vi "FindStartEndPointsRRTImproved.vi"(4 "ignoreBall?":bool, 5 "Robot in":T1={"id"=0, "function"=enum."Attacker", "x"=0.0, "y"=0.0, "orientation"=0.0, "v_tangent"=0.0, "v_normal"=0.0, "v_ang"=0.0, "kick_x"=0.0, "kick_z"=0.0, "dribble"=FALSE, "Timestamp"=timestamp(0 s since 1904-01-01), "estimatives"={"est_v_tangent"=0.0, "est_v_normal"=0.0, "est_vx"=0.0, "est_vy"=0.0, "Pos Robot Est"=[]}, "dest_x_kick"=0.0, "dest_y_kick"=0.0, "Gap Coord"=[], "States"=enum."Pass", "Path "=[], "Path  Smooth"=[], "Dest"=[], "vx_desired"=0.0, "vy_desired"=0.0, "slowBehavior"=FALSE, "VSSStates"=enum."Pass"}, 6 "enemy_robots":T1[](array[typedef]), 7 "ball":dbl[](array[numeric]), 8 "our_robots":T1[](array[typedef]), 9 "Goal":dbl[](array[numeric]), 10 "Initial State":dbl[](array[numeric]), 11 "Collision Points":dbl[][](array[numeric])) -> (2 "Start End Points RRT":dbl[][](array[numeric]))   [LabVIEW 2020]
uses:
  Vision_class/Old vision/Controls/AI Robot.ctl
  Vision_class/Old vision/Controls/Functions Enum.ctl
  Vision_class/Old vision/Controls/AttackerStates.ctl
  Vision_class/Old vision/Controls/PathDests.ctl
  Vision_class/Old vision/Controls/PathDest.ctl
  Navigation/VSSNavigation/VSSAttackerStates.ctl
  <vilib>/Analysis/_algsub.llb/Real Vector Norm.vi
  <vilib>/Analysis/NI_AALPro.lvlib
panel:
  in  "tamanho minimo":dbl=300.0 format="%#_13g"
  in  "threshold":dbl=100.0 format="%#_13g"
  out "Collision Points \nordenado":dbl[][](array[numeric])
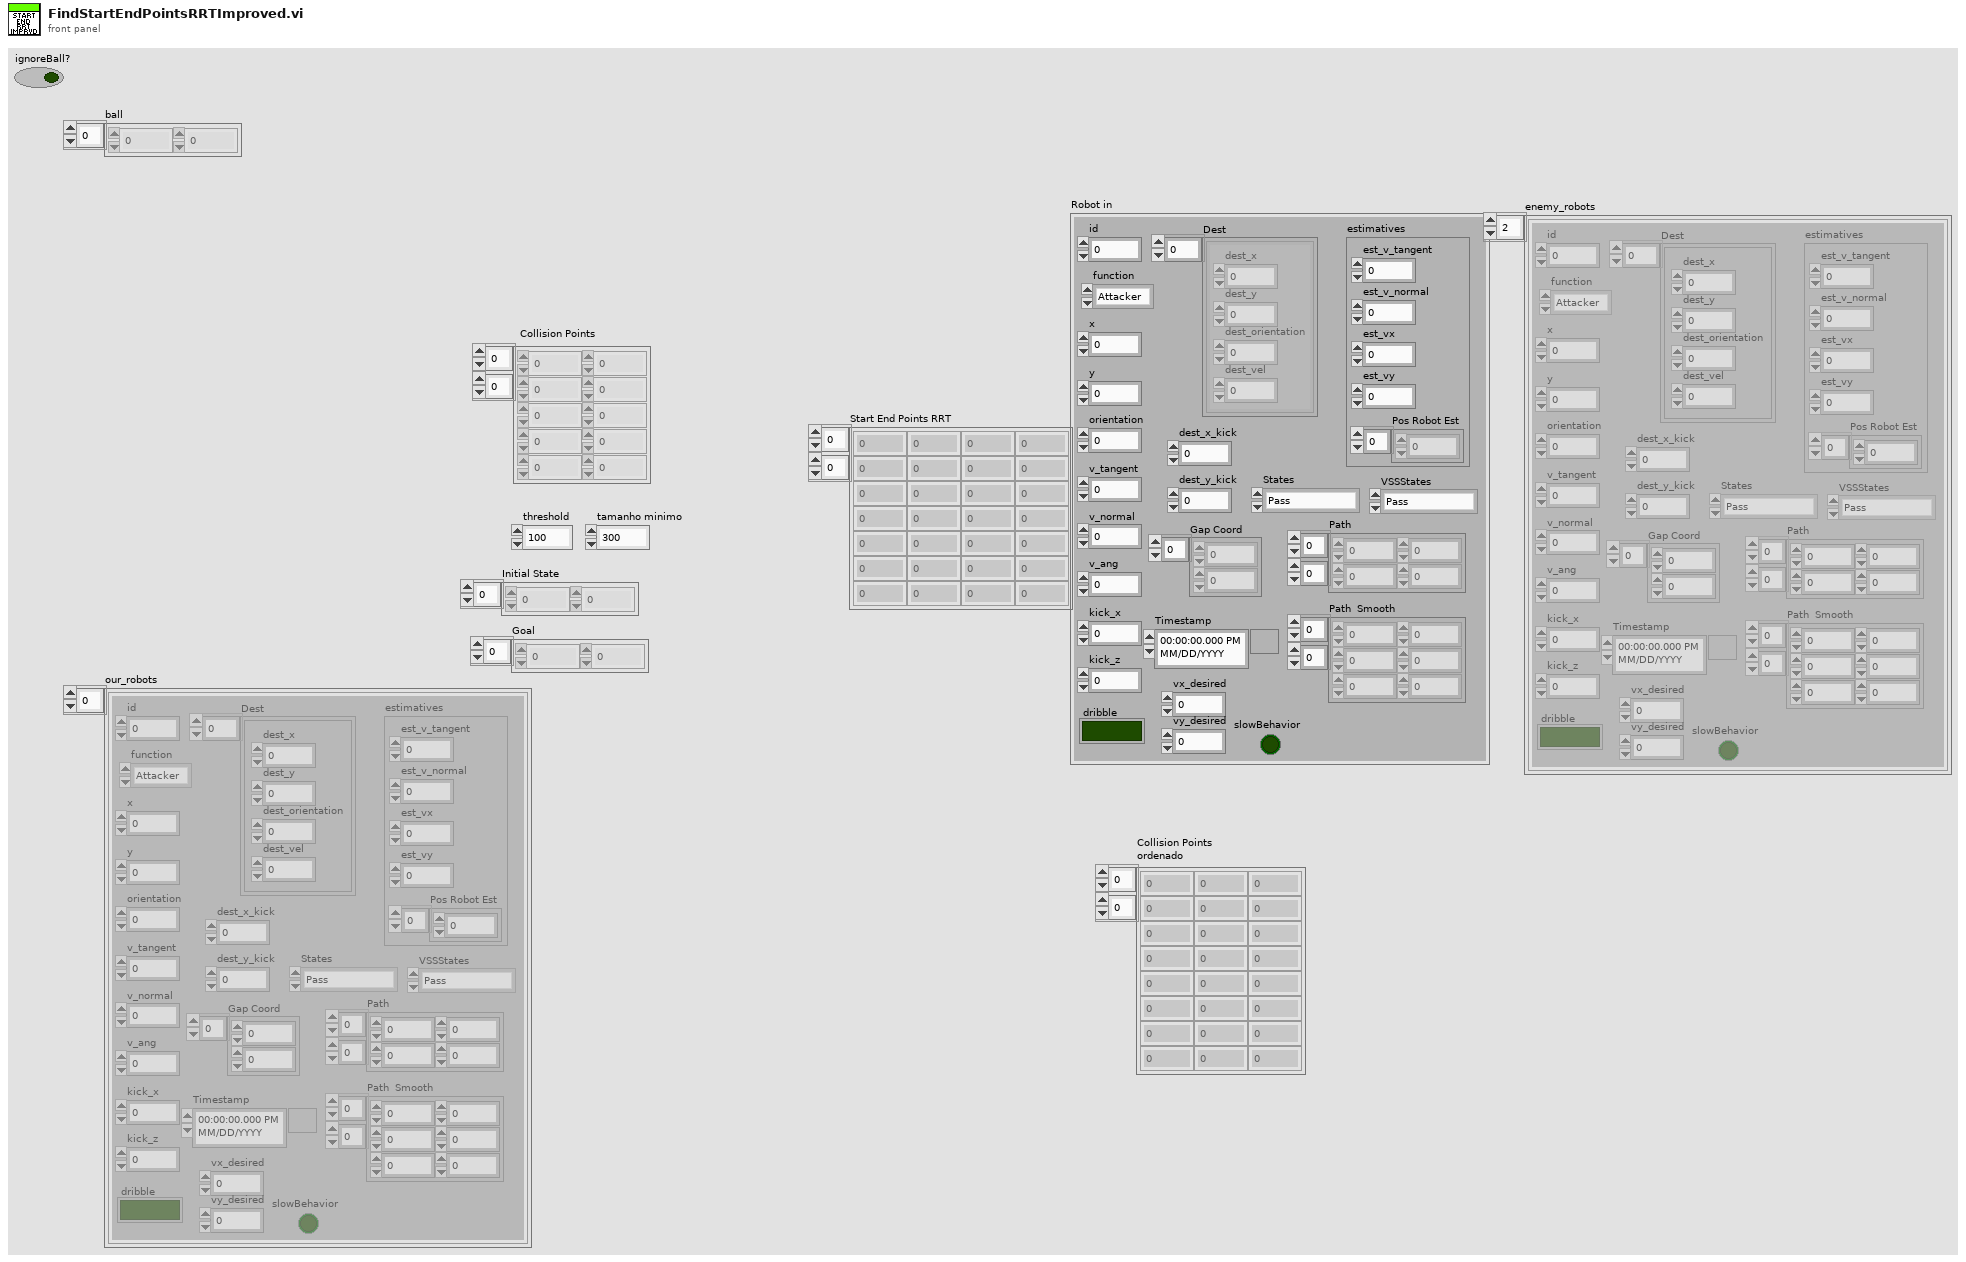
[diagram p1: front panel]
types:
  T1 = typedef "AI Robot.ctl" = cluster{"id":u32, "function":T2, "x":dbl, "y":dbl, "orientation":dbl, "v_tangent":dbl, "v_normal":dbl, "v_ang":dbl, "kick_x":dbl, "kick_z":dbl, "dribble":bool, "Timestamp":timestamp, "estimatives":cluster{"est_v_tangent":dbl, "est_v_normal":dbl, "est_vx":dbl, "est_vy":dbl, "Pos Robot Est":dbl[]}, "dest_x_kick":dbl, "dest_y_kick":dbl, "Gap Coord":dbl[], "States":T3, "Path ":dbl[][], "Path  Smooth":dbl[][], "Dest":T4, "vx_desired":dbl, "vy_desired":dbl, "slowBehavior":bool, "VSSStates":T6}
  T2 = typedef "Functions Enum.ctl" = enum16{"2nd Striker", "Attacker", "Goalie", "Defender", "Striker", "Goto 0", "Dummy", "Kicker", "ZigZag 0", "ZigZag 1", "ZigZag 2", "ZigZag 3", "ZigZag 4", "ZigZag 5", "ZigZag 6", "ZigZag 7", "ZigZag 8", ""}
  T3 = typedef "AttackerStates.ctl" = enum16{"Pass", "GoToTangent", "BallGetting", "GoToKick", ""}
  T4 = typedef "PathDests.ctl" = T5[]
  T5 = typedef "PathDest.ctl" = cluster{"dest_x":dbl, "dest_y":dbl, "dest_orientation":dbl, "dest_vel":dbl}
  T6 = typedef "VSSAttackerStates.ctl" = enum16{"Pass", "GoToTangent", "BallGetting", "GoToKick", "Rotate anti-clockwise", "Rotate Clockwise", ""}
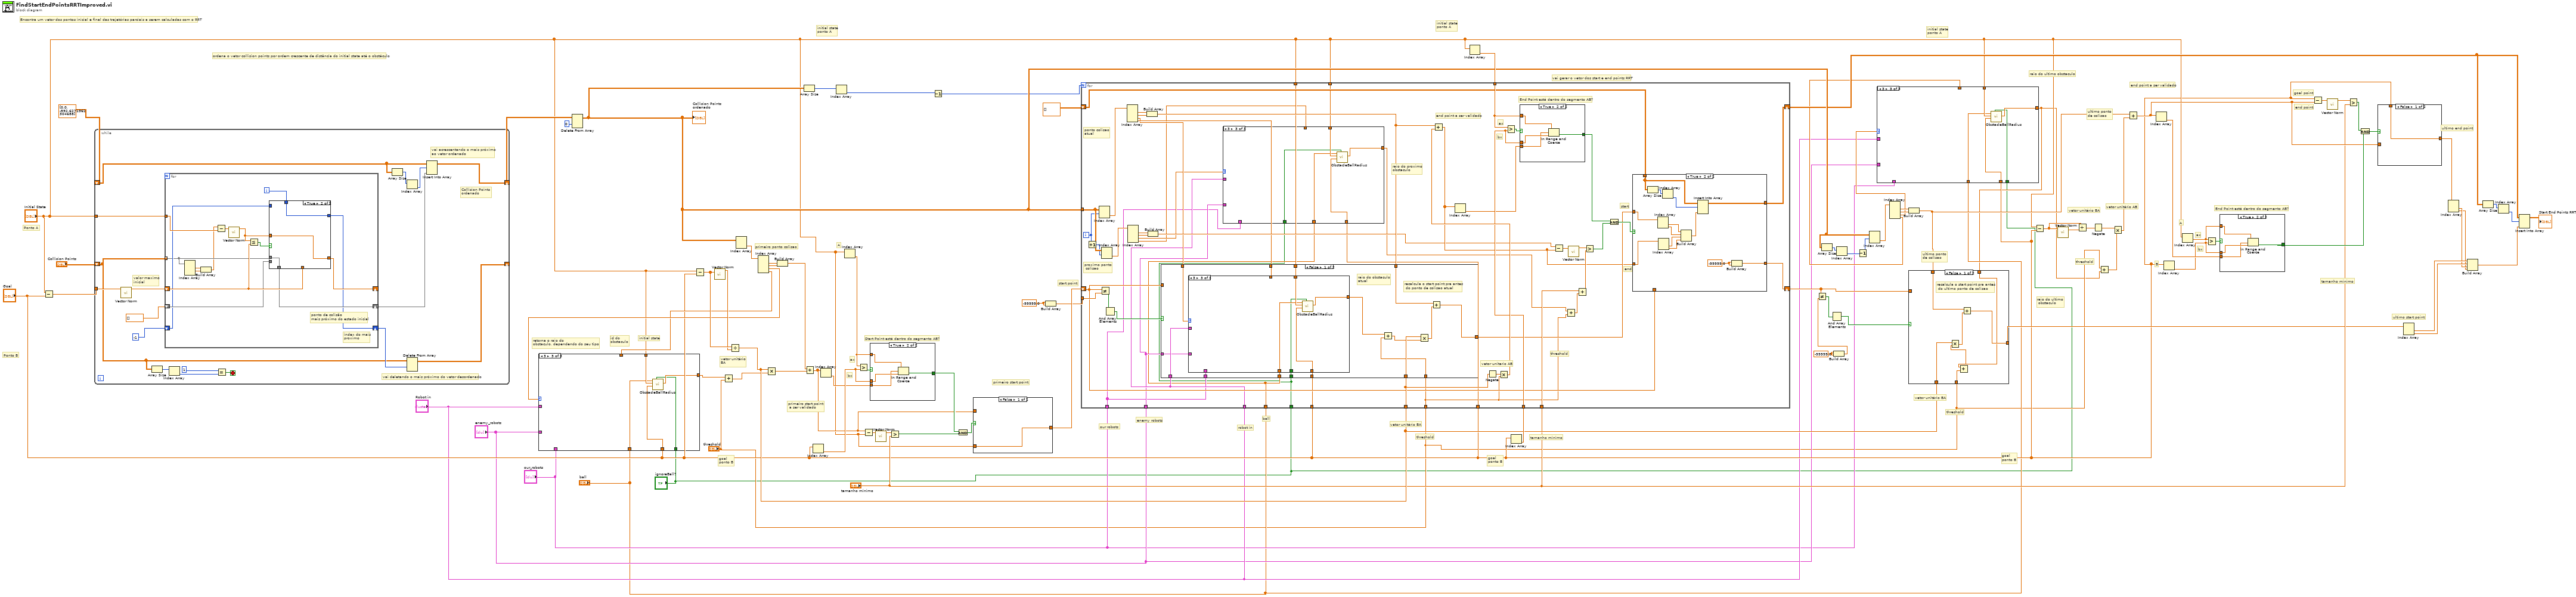
[diagram p0: block diagram]
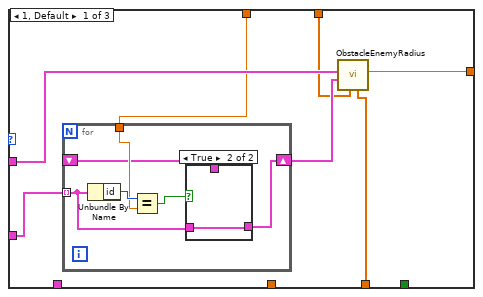
[diagram p2: hidden frame]
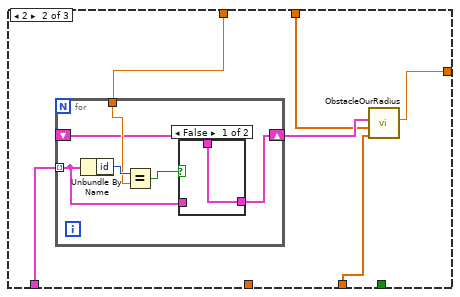
[diagram p4: hidden frame]
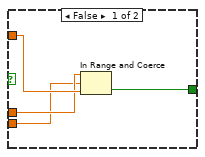
[diagram p6: hidden frame]
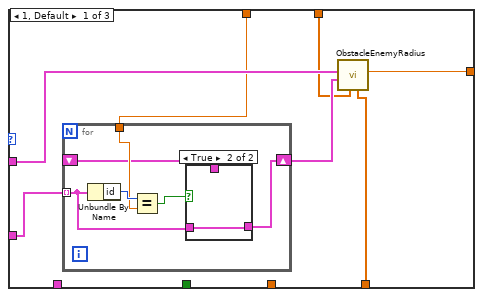
[diagram p9: hidden frame]
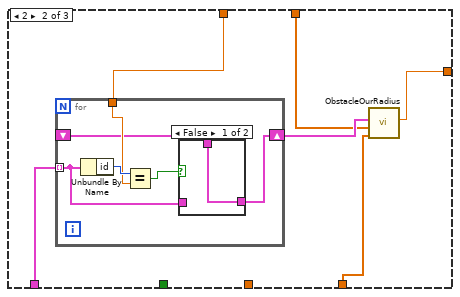
[diagram p11: hidden frame]
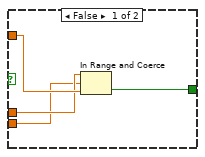
[diagram p14: hidden frame]
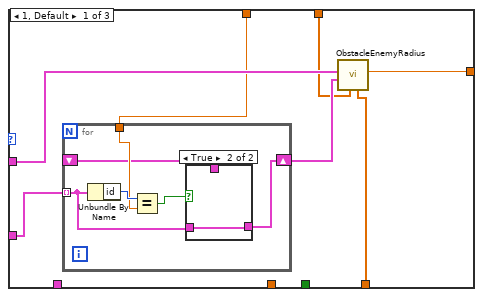
[diagram p15: hidden frame]
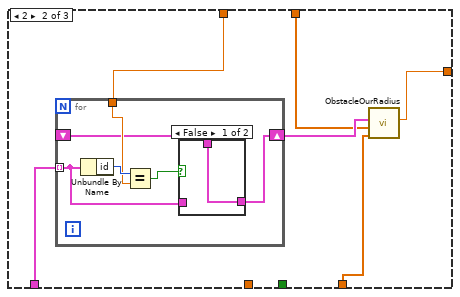
[diagram p17: hidden frame]
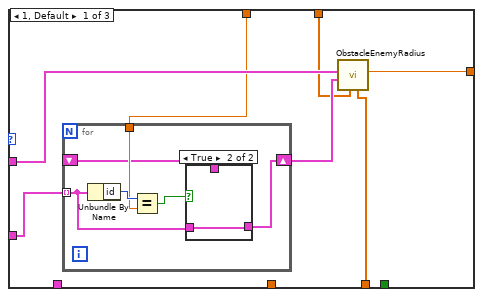
[diagram p20: hidden frame]
diagram:
  w47 = -99999.0 ("element")
  w52 = -99999.0 ("element")
  # "raio do ultimo\n obstaculo"
  # "raio do ultimo obstaculo"
  # "ball"
  # "robot in"
  # "enemy robots"
  # "our robots"
  # "initial state"
  # "id do\nobstaculo"
  # "retorna o raio do \nobstaculo, dependendo do seu tipo"
  # "vai gerar o vetor dos start e end points RRT"
  # "ultimo start point"
  # "ultimo end point"
  # "tamanho minimo"
  # "end point a ser validado"
  # "ultimo ponto\nde colisao"
  # "threshold"
  # "goal\nponto B"
  # "initial state\nponto A"
  # "ultimo ponto\nde colisao"
  # "threshold"
  # "vetor unitário BA"
  # "tamanho minimo"
  # "initial state\nponto A"
  # "goal\nponto B"
  # "threshold"
  # "vetor unitário BA"
  # "start point"
  # "primeiro start point"
  # "A"
  # "Start Point está dentro do segmento AB?"
  # "bx"
  # "ax"
  # "primeiro start point\n a ser validado"
  # "primeiro ponto colisao"
  # "vetor unitário\nBA"
  # "initial state\nponto A"
  # "goal\nponto B"
  # "ordena o vetor collision points por ordem crescente de distância do initial state até o obstáculo"
  # "Encontra um vetor dos pontos inicial e final das trajetórias parciais a serem calculadas com o RRT"
  # "end point"
  # "goal point"
  # "End Point está dentro do segmento AB?"
  # "bx"
  # "ax"
  # "B"
  # "A"
  # "vetor unitário AB"
  # "vetor unitário BA"
  # "Ponto B"
  # "Ponto A"
  n1 = Subtract(x="Initial State", y="Goal") -> (x-y=w88:dbl[])
  n2 = while {
    tunnel: w88 -> [w105]
    tunnel: "Initial State" -> [w102]
    shift-right: [w98] -> w69
    shift-left: dbl[][] [[0.0, -592.6271362304688]] ("Collision Points") -> [w100]
    shift-right: [w94] -> _
    shift-left: "Collision Points" -> [w93]
    stop <- w90 stop-if-true
    # "vai acrescentando o mais próximo\nao vetor ordenado"
    # "vai deletando o mais próximo do vetor desordenado"
    # "Collision Points \nordenado"
    # "valor maximo\ninicial"
    n3 = call-poly <vilib>:"Vector Norm.vi"("Input Vector"=w105) -> ("norm"=w104:dbl)  [unwired: 9 in, 1 out]
    n4 = Array Size(array=w93) -> (size(s)=w92:i32[])
    n5 = for {
      tunnel: w93 -> [w109] mode=indexing
      tunnel: w102 -> [w113]
      shift-right: [w117] -> _
      shift-left: w104 -> [w118]
      shift-right: [w116] -> w99
      shift-left: dbl[] [] ("Goal 2") -> [w115]
      shift-right: [w111] -> w95
      shift-left: -1 -> [w110]
      i -> [w112]
      # "index do mais\nproximo"
      # "ponto de colisão \nmais próximo do estado inicial"
      n6 = Index Array(array=w109) -> (element #1=w108:dbl, element #2=w107:dbl)  [unwired: 3 in, 1 out]
      n7 = Build Array(w108, w107) -> (w106:dbl[])
      n8 = Subtract(x=w106, y=w113) -> (x-y=w120:dbl[])
      n9 = call-poly <vilib>:"Vector Norm.vi"("Input Vector"=w120) -> ("norm"=w114:dbl)  [unwired: 9 in, 1 out]
      n10 = Less Or Equal?(x=w114, y=w118) -> (x <= y?=w119:bool)
      n11 = case shown="True" w119 {
        tunnel: [w123 w126] -> w117
        tunnel: w114 -> [_ w126]
        tunnel: w118 -> [w123 _]
        tunnel: w109 -> [_ w125]
        tunnel: [w122 w125] -> w116
        tunnel: w115 -> [w122 _]
        tunnel: w112 -> [_ w124]
        tunnel: [w121 w124] -> w111
        tunnel: w110 -> [w121 _]
        frame False {
        }
        frame True {
        }
      }
    }
    n12 = Index Array(array=w92) -> (element=w91:i32)  [unwired: 1 in]
    n13 = Equal?(x=1, y=w91) -> (x = y?=w90:bool)
    n14 = Array Size(array=w100) -> (size(s)=w97:i32[])
    n15 = Index Array(array=w97) -> (element=w96:i32)  [unwired: 1 in]
    n16 = Delete From Array(array=w93, index (row)=w95) -> (array with subset deleted=w94:dbl[][])  [unwired: 2 in, 1 out]
    n17 = Insert Into Array(array=w100, index (row)=w96, new element=w99) -> (w98:dbl[][])  [unwired: 1 in]
  }
  n18 = Delete From Array(array=w69, index (row)=0) -> (array with subset deleted=w42:dbl[][])  [unwired: 2 in, 1 out]
  "Collision Points \nordenado" <- w42
  n19 = Subtract(x="Initial State", y="Goal") -> (x-y=w66:dbl[])
  n20 = call-poly <vilib>:"Vector Norm.vi"("Input Vector"=w66) -> ("norm"=w65:dbl)  [unwired: 9 in, 1 out]
  n21 = Divide(x=w66, y=w65) -> (x/y=w48:dbl[])
  n22 = Index Array(array=w42) -> (element=w22:dbl[])  [unwired: 2 in]
  n23 = Index Array(array=w22) -> (element #1=w24:dbl, element #2=w23:dbl, element #3=w20:dbl, element #4=w19:dbl)  [unwired: 4 in]
  n24 = case shown="3" w20 {
    tunnel: "Robot in" -> [w133 _ _]
    tunnel: "enemy_robots" -> [w132 _ _]
    tunnel: w19 -> [w131 w146 _]
    tunnel: "Goal" -> [w129 w143 w159]
    tunnel: "Initial State" -> [w128 w144 w160]
    tunnel: [w127 w142 w158] -> w17
    tunnel: "our_robots" -> [_ w147 _]
    tunnel: "ball" -> [_ _ w157]
    tunnel: "ignoreBall?" -> [_ _ w156]
    frame 1, Default {
      n25 = for {
        tunnel: w132 -> [w136] mode=indexing
        shift-right: [w135] -> w130
        shift-left: _ -> [w134]
        tunnel: w131 -> [w138]
        n26 = Unbundle By Name(w136) -> ("id"=w139:u32)
        n27 = Equal?(x=w139, y=w138) -> (x = y?=w137:bool)
        n28 = case shown="True" w137 {
          tunnel: w136 -> [_ w141]
          tunnel: [w140 w141] -> w135
          tunnel: w134 -> [w140 _]
          frame False {
          }
          frame True {
          }
        }
      }
      n29 = call "ObstacleEnemyRadius.vi"("Goal"=w129, "Initial State"=w128, "Robot enemy"=w130, "Robot in"=w133) -> ("obstacle enemy radius"=w127:dbl)  [unwired: 7 in]
    }
    frame 2 {
      n30 = for {
        tunnel: w147 -> [w150] mode=indexing
        shift-right: [w149] -> w145
        shift-left: _ -> [w148]
        tunnel: w146 -> [w152]
        n31 = Unbundle By Name(w150) -> ("id"=w153:u32)
        n32 = Equal?(x=w153, y=w152) -> (x = y?=w151:bool)
        n33 = case shown="False" w151 {
          tunnel: w150 -> [_ w155]
          tunnel: [w154 w155] -> w149
          tunnel: w148 -> [w154 _]
          frame False {
          }
          frame True {
          }
        }
      }
      n34 = call "ObstacleOurRadius.vi"("Goal"=w143, "Initial State"=w144, "other robot"=w145) -> ("obstacle enemy radius"=w142:dbl)  [unwired: 8 in]
    }
    frame 3 {
      n35 = call "ObstacleBallRadius.vi"("ignoreBall?"=w156, "Goal"=w159, "Initial State"=w160, "ball"=w157) -> ("obstacle enemy radius"=w158:dbl)  [unwired: 7 in]
    }
  }
  n36 = Add(x=w17, y="threshold") -> (x+y=w18:dbl)
  n37 = Multiply(x=w48, y=w18) -> (x*y=w64:dbl[])
  n38 = Build Array(w24, w23) -> (w21:dbl[])
  n39 = Array Size(array=w42) -> (size(s)=w68:i32[])
  n40 = Add(x=w21, y=w64) -> (x+y=w54:dbl[])
  n41 = Index Array(array="Goal") -> (element=w61:dbl)  [unwired: 1 in]
  n42 = Index Array(array=w54) -> (element=w60:dbl)  [unwired: 1 in]
  n43 = Index Array(array=w68) -> (element=w67:i32)  [unwired: 1 in]
  n44 = Index Array(array="Initial State") -> (element=w62:dbl)  [unwired: 1 in]
  n45 = Greater?(x=w62, y=w61) -> (0:w63:bool)
  n46 = Subtract(x=w54, y="Initial State") -> (x-y=w59:dbl[])
  n47 = case shown="True" w63 {
    tunnel: w62 -> [w164 w168]
    tunnel: w61 -> [w163 w167]
    tunnel: w60 -> [w162 w166]
    tunnel: [w161 w165] -> w57
    frame False {
      n48 = In Range and Coerce(upper limit=w163, x=w162, lower limit=w164) -> (In Range?=w161:bool)  [unwired: 1 out]
    }
    frame True {
      n49 = In Range and Coerce(upper limit=w168, x=w166, lower limit=w167) -> (In Range?=w165:bool)  [unwired: 1 out]
    }
  }
  n50 = call-poly <vilib>:"Vector Norm.vi"("Input Vector"=w59) -> ("norm"=w58:dbl)  [unwired: 9 in, 1 out]
  n51 = Greater?(x=w58, y="tamanho minimo") -> (0:w56:bool)
  n52 = Decrement(x=w67) -> (x-1=w27:i32)
  n53 = And(x=w57, y=w56) -> (x .and. y?=w55:bool)
  n54 = case shown="False" w55 {
    tunnel: [w169 w170] -> w53
    tunnel: w54 -> [_ w170]
    tunnel: "Initial State" -> [w169 _]
    frame False {
    }
    frame True {
    }
  }
  n55 = Build Array(w52, w52) -> (w51:dbl[])
  n56 = Index Array(array="Initial State") -> (element=w50:dbl)  [unwired: 1 in]
  n57 = Index Array(array="Goal") -> (element=w49:dbl)  [unwired: 1 in]
  n58 = for {
    N: w27 -> [_]
    tunnel: w42 -> [w220]
    shift-right: [w198] -> w25
    shift-left: dbl[][] [] -> [w201]
    shift-right: [w197] -> w43
    shift-left: w53 -> [w195]
    tunnel: w51 -> [w217]
    tunnel: w48 -> [w215]
    tunnel: "threshold" -> [w174]
    tunnel: w50 -> [w211]
    tunnel: w49 -> [w210]
    tunnel: "tamanho minimo" -> [w207]
    tunnel: "Initial State" -> [w185]
    tunnel: "our_robots" -> [w176]
    tunnel: "enemy_robots" -> [w179]
    tunnel: "Robot in" -> [w180]
    tunnel: "Goal" -> [w183]
    tunnel: "ball" -> [w175]
    tunnel: "Initial State" -> [w182]
    tunnel: "Goal" -> [w181]
    tunnel: "ignoreBall?" -> [w171]
    i -> [w219]
    # "raio do proximo\nobstaculo"
    # "end"
    # "start"
    # "threshold"
    # "End Point está dentro do segmento AB?"
    # "bx"
    # "ax"
    # "end point a ser validado"
    # "vetor unitario AB"
    # "proximo ponto\n colisao"
    # "ponto colisao\natual"
    n59 = Increment(x=w219) -> (x+1=w218:i32)
    n60 = Index Array(array=w220, index (row)=w219) -> (element=w192:dbl[])  [unwired: 1 in]
    n61 = Not Equal?(x=w195, y=w217) -> (x != y?=w216:bool[])
    n62 = Index Array(array=w220, index (row)=w218) -> (element=w188:dbl[])  [unwired: 1 in]
    n63 = And Array Elements(Boolean array=w216) -> (logical AND=w196:bool)
    n64 = Index Array(array=w192) -> (element #1=w194:dbl, element #2=w193:dbl, element #3=w184:dbl, element #4=w186:dbl)  [unwired: 4 in]
    n65 = Index Array(array=w188) -> (element #1=w189:dbl, element #2=w190:dbl, element #3=w178:dbl, element #4=w177:dbl)  [unwired: 4 in]
    n66 = Build Array(w194, w193) -> (w191:dbl[])
    n67 = Build Array(w189, w190) -> (w187:dbl[])
    n68 = case shown="False" w196 {
      tunnel: w195 -> [_ w328]
      tunnel: [w290 w328] -> w200
      tunnel: w215 -> [w293 _]
      tunnel: w174 -> [w286 _]
      tunnel: w191 -> [w292 _]
      tunnel: w186 -> [w289 _]
      tunnel: w185 -> [w288 _]
      tunnel: w184 -> [w284 _]
      tunnel: w180 -> [w283 _]
      tunnel: w179 -> [w282 _]
      tunnel: w183 -> [w281 _]
      tunnel: w176 -> [w280 _]
      tunnel: w175 -> [w279 _]
      tunnel: w171 -> [w278 _]
      frame False {
        # "raio do obstaculo\natual"
        # "recalcula o start point pra antes\n do ponto de colisao atual"
        n69 = case shown="3" w284 {
          tunnel: w283 -> [w300 _ _]
          tunnel: w282 -> [w299 _ _]
          tunnel: w289 -> [w298 w313 _]
          tunnel: w281 -> [w296 w310 w326]
          tunnel: w288 -> [w295 w311 w327]
          tunnel: [w294 w309 w325] -> w287
          tunnel: w280 -> [_ w314 _]
          tunnel: w279 -> [_ _ w324]
          tunnel: w278 -> [_ _ w323]
          frame 1, Default {
            n70 = for {
              tunnel: w299 -> [w303] mode=indexing
              shift-right: [w302] -> w297
              shift-left: _ -> [w301]
              tunnel: w298 -> [w305]
              n71 = Unbundle By Name(w303) -> ("id"=w306:u32)
              n72 = Equal?(x=w306, y=w305) -> (x = y?=w304:bool)
              n73 = case shown="True" w304 {
                tunnel: w303 -> [_ w308]
                tunnel: [w307 w308] -> w302
                tunnel: w301 -> [w307 _]
                frame False {
                }
                frame True {
                }
              }
            }
            n74 = call "ObstacleEnemyRadius.vi"("Goal"=w296, "Initial State"=w295, "Robot enemy"=w297, "Robot in"=w300) -> ("obstacle enemy radius"=w294:dbl)  [unwired: 7 in]
          }
          frame 2 {
            n75 = for {
              tunnel: w314 -> [w317] mode=indexing
              shift-right: [w316] -> w312
              shift-left: _ -> [w315]
              tunnel: w313 -> [w319]
              n76 = Unbundle By Name(w317) -> ("id"=w320:u32)
              n77 = Equal?(x=w320, y=w319) -> (x = y?=w318:bool)
              n78 = case shown="False" w318 {
                tunnel: w317 -> [_ w322]
                tunnel: [w321 w322] -> w316
                tunnel: w315 -> [w321 _]
                frame False {
                }
                frame True {
                }
              }
            }
            n79 = call "ObstacleOurRadius.vi"("Goal"=w310, "Initial State"=w311, "other robot"=w312) -> ("obstacle enemy radius"=w309:dbl)  [unwired: 8 in]
          }
          frame 3 {
            n80 = call "ObstacleBallRadius.vi"("ignoreBall?"=w323, "Goal"=w326, "Initial State"=w327, "ball"=w324) -> ("obstacle enemy radius"=w325:dbl)  [unwired: 7 in]
          }
        }
        n81 = Add(x=w287, y=w286) -> (x+y=w285:dbl)
        n82 = Multiply(x=w293, y=w285) -> (x*y=w291:dbl[])
        n83 = Add(x=w292, y=w291) -> (x+y=w290:dbl[])
      }
      frame True {
        # "start  point ainda é valido, \ne nao precisa recalcular"
      }
    }
    n84 = case shown="3" w178 {
      tunnel: w180 -> [w227 _ _]
      tunnel: w179 -> [w226 _ _]
      tunnel: w177 -> [w225 w240 _]
      tunnel: w181 -> [w223 w237 w253]
      tunnel: w182 -> [w222 w238 w254]
      tunnel: [w221 w236 w252] -> w173
      tunnel: w176 -> [_ w241 _]
      tunnel: w175 -> [_ _ w251]
      tunnel: w171 -> [_ _ w250]
      frame 1, Default {
        n85 = for {
          tunnel: w226 -> [w230] mode=indexing
          shift-right: [w229] -> w224
          shift-left: _ -> [w228]
          tunnel: w225 -> [w232]
          n86 = Unbundle By Name(w230) -> ("id"=w233:u32)
          n87 = Equal?(x=w233, y=w232) -> (x = y?=w231:bool)
          n88 = case shown="True" w231 {
            tunnel: w230 -> [_ w235]
            tunnel: [w234 w235] -> w229
            tunnel: w228 -> [w234 _]
            frame False {
            }
            frame True {
            }
          }
        }
        n89 = call "ObstacleEnemyRadius.vi"("Goal"=w223, "Initial State"=w222, "Robot enemy"=w224, "Robot in"=w227) -> ("obstacle enemy radius"=w221:dbl)  [unwired: 7 in]
      }
      frame 2 {
        n90 = for {
          tunnel: w241 -> [w244] mode=indexing
          shift-right: [w243] -> w239
          shift-left: _ -> [w242]
          tunnel: w240 -> [w246]
          n91 = Unbundle By Name(w244) -> ("id"=w247:u32)
          n92 = Equal?(x=w247, y=w246) -> (x = y?=w245:bool)
          n93 = case shown="False" w245 {
            tunnel: w244 -> [_ w249]
            tunnel: [w248 w249] -> w243
            tunnel: w242 -> [w248 _]
            frame False {
            }
            frame True {
            }
          }
        }
        n94 = call "ObstacleOurRadius.vi"("Goal"=w237, "Initial State"=w238, "other robot"=w239) -> ("obstacle enemy radius"=w236:dbl)  [unwired: 8 in]
      }
      frame 3 {
        n95 = call "ObstacleBallRadius.vi"("ignoreBall?"=w250, "Goal"=w253, "Initial State"=w254, "ball"=w251) -> ("obstacle enemy radius"=w252:dbl)  [unwired: 7 in]
      }
    }
    n96 = Negate(x=w215) -> (-x=w214:dbl[])
    n97 = Multiply(x=w214, y=w174) -> (x*y=w213:dbl[])
    n98 = Add(x=w191, y=w213) -> (x+y=w199:dbl[])
    n99 = Index Array(array=w199) -> (element=w203:dbl)  [unwired: 1 in]
    n100 = Greater?(x=w211, y=w210) -> (0:w212:bool)
    n101 = case shown="True" w212 {
      tunnel: w211 -> [w273 w277]
      tunnel: w210 -> [w272 w276]
      tunnel: w203 -> [w271 w275]
      tunnel: [w270 w274] -> w205
      frame False {
        n102 = In Range and Coerce(upper limit=w272, x=w271, lower limit=w273) -> (In Range?=w270:bool)  [unwired: 1 out]
      }
      frame True {
        n103 = In Range and Coerce(upper limit=w277, x=w275, lower limit=w276) -> (In Range?=w274:bool)  [unwired: 1 out]
      }
    }
    n104 = Subtract(x=w187, y=w199) -> (x-y=w209:dbl[])
    n105 = Add(x=w173, y=w174) -> (x+y=w172:dbl)
    n106 = call-poly <vilib>:"Vector Norm.vi"("Input Vector"=w209) -> ("norm"=w208:dbl)  [unwired: 9 in, 1 out]
    n107 = Add(x=w207, y=w172) -> (x+y=w206:dbl)
    n108 = Greater?(x=w208, y=w206) -> (0:w204:bool)
    n109 = And(x=w205, y=w204) -> (x .and. y?=w202:bool)
    n110 = case shown="True" w202 {
      tunnel: w201 -> [w256 w268]
      tunnel: w200 -> [_ w266]
      tunnel: w199 -> [_ w265]
      tunnel: [w256 w259] -> w198
      tunnel: [w255 w257] -> w197
      tunnel: w195 -> [w255 _]
      frame False {
      }
      frame True {
        w258 = -99999.0 ("element")
        n111 = Array Size(array=w268) -> (size(s)=w269:i32[])
        n112 = Index Array(array=w266) -> (element #1=w264:dbl, element #2=w263:dbl)  [unwired: 2 in]
        n113 = Index Array(array=w265) -> (element #1=w262:dbl, element #2=w261:dbl)  [unwired: 2 in]
        n114 = Index Array(array=w269) -> (element=w267:i32)  [unwired: 1 in]
        n115 = Build Array(w264, w263, w262, w261) -> (w260:dbl[])
        n116 = Insert Into Array(array=w268, index (row)=w267, new element=w260) -> (w259:dbl[][])  [unwired: 1 in]
        n117 = Build Array(w258, w258) -> (w257:dbl[])
      }
    }
  }
  n118 = Array Size(array=w42) -> (size(s)=w41:i32[])
  n119 = Build Array(w47, w47) -> (w46:dbl[])
  n120 = Not Equal?(x=w43, y=w46) -> (x != y?=w45:bool[])
  n121 = And Array Elements(Boolean array=w45) -> (logical AND=w44:bool)
  n122 = Index Array(array=w41) -> (element=w40:i32)  [unwired: 1 in]
  n123 = Decrement(x=w40) -> (x-1=w39:i32)
  n124 = Index Array(array=w42, index (row)=w39) -> (element=w14:dbl[])  [unwired: 1 in]
  n125 = Index Array(array=w14) -> (element #1=w16:dbl, element #2=w15:dbl, element #3=w12:dbl, element #4=w11:dbl)  [unwired: 4 in]
  n126 = case shown="3" w12 {
    tunnel: "Robot in" -> [w335 _ _]
    tunnel: "enemy_robots" -> [w334 _ _]
    tunnel: w11 -> [w333 w348 _]
    tunnel: "Goal" -> [w331 w345 w361]
    tunnel: "Initial State" -> [w330 w346 w362]
    tunnel: [w329 w344 w360] -> w2
    tunnel: "our_robots" -> [_ w349 _]
    tunnel: "ball" -> [_ _ w359]
    tunnel: "ignoreBall?" -> [_ _ w358]
    frame 1, Default {
      n127 = for {
        tunnel: w334 -> [w338] mode=indexing
        shift-right: [w337] -> w332
        shift-left: _ -> [w336]
        tunnel: w333 -> [w340]
        n128 = Unbundle By Name(w338) -> ("id"=w341:u32)
        n129 = Equal?(x=w341, y=w340) -> (x = y?=w339:bool)
        n130 = case shown="True" w339 {
          tunnel: w338 -> [_ w343]
          tunnel: [w342 w343] -> w337
          tunnel: w336 -> [w342 _]
          frame False {
          }
          frame True {
          }
        }
      }
      n131 = call "ObstacleEnemyRadius.vi"("Goal"=w331, "Initial State"=w330, "Robot enemy"=w332, "Robot in"=w335) -> ("obstacle enemy radius"=w329:dbl)  [unwired: 7 in]
    }
    frame 2 {
      n132 = for {
        tunnel: w349 -> [w352] mode=indexing
        shift-right: [w351] -> w347
        shift-left: _ -> [w350]
        tunnel: w348 -> [w354]
        n133 = Unbundle By Name(w352) -> ("id"=w355:u32)
        n134 = Equal?(x=w355, y=w354) -> (x = y?=w353:bool)
        n135 = case shown="False" w353 {
          tunnel: w352 -> [_ w357]
          tunnel: [w356 w357] -> w351
          tunnel: w350 -> [w356 _]
          frame False {
          }
          frame True {
          }
        }
      }
      n136 = call "ObstacleOurRadius.vi"("Goal"=w345, "Initial State"=w346, "other robot"=w347) -> ("obstacle enemy radius"=w344:dbl)  [unwired: 8 in]
    }
    frame 3 {
      n137 = call "ObstacleBallRadius.vi"("ignoreBall?"=w358, "Goal"=w361, "Initial State"=w362, "ball"=w359) -> ("obstacle enemy radius"=w360:dbl)  [unwired: 7 in]
    }
  }
  n138 = Build Array(w16, w15) -> (w13:dbl[])
  n139 = case shown="False" w44 {
    tunnel: w43 -> [_ w370]
    tunnel: [w367 w370] -> w36
    tunnel: w48 -> [w369 _]
    tunnel: "threshold" -> [w365 _]
    tunnel: w13 -> [w366 _]
    tunnel: w2 -> [w364 _]
    frame False {
      # "recalcula o start point pra antes\n do ultimo ponto de colisao"
      n140 = Add(x=w364, y=w365) -> (x+y=w363:dbl)
      n141 = Multiply(x=w369, y=w363) -> (x*y=w368:dbl[])
      n142 = Add(x=w366, y=w368) -> (x+y=w367:dbl[])
    }
    frame True {
      # "start  point ainda é valido, \ne nao precisa recalcular"
    }
  }
  n143 = Subtract(x="Initial State", y="Goal") -> (x-y=w87:dbl[])
  n144 = call-poly <vilib>:"Vector Norm.vi"("Input Vector"=w87) -> ("norm"=w86:dbl)  [unwired: 9 in, 1 out]
  n145 = Divide(x=w87, y=w86) -> (x/y=w83:dbl[])
  n146 = Negate(x=w83) -> (-x=w85:dbl[])
  n147 = Add(x="threshold", y=w2) -> (x+y=w3:dbl)
  n148 = Multiply(x=w85, y=w3) -> (x*y=w84:dbl[])
  n149 = Add(x=w13, y=w84) -> (x+y=w73:dbl[])
  n150 = Index Array(array=w73) -> (element=w82:dbl)  [unwired: 1 in]
  n151 = Index Array(array="Goal") -> (element=w80:dbl)  [unwired: 1 in]
  n152 = Index Array(array="Initial State") -> (element=w79:dbl)  [unwired: 1 in]
  n153 = Greater?(x=w79, y=w80) -> (0:w81:bool)
  n154 = case shown="True" w81 {
    tunnel: w79 -> [w374 w378]
    tunnel: w80 -> [w373 w377]
    tunnel: w82 -> [w372 w376]
    tunnel: [w371 w375] -> w76
    frame False {
      n155 = In Range and Coerce(upper limit=w373, x=w372, lower limit=w374) -> (In Range?=w371:bool)  [unwired: 1 out]
    }
    frame True {
      n156 = In Range and Coerce(upper limit=w378, x=w376, lower limit=w377) -> (In Range?=w375:bool)  [unwired: 1 out]
    }
  }
  n157 = Subtract(x="Goal", y=w73) -> (x-y=w78:dbl[])
  n158 = call-poly <vilib>:"Vector Norm.vi"("Input Vector"=w78) -> ("norm"=w77:dbl)  [unwired: 9 in, 1 out]
  n159 = Greater?(x=w77, y="tamanho minimo") -> (0:w75:bool)
  n160 = And(x=w75, y=w76) -> (x .and. y?=w74:bool)
  n161 = case shown="False" w74 {
    tunnel: w73 -> [_ w380]
    tunnel: [w379 w380] -> w37
    tunnel: "Goal" -> [w379 _]
    frame False {
    }
    frame True {
    }
  }
  n162 = Index Array(array=w36) -> (element #1=w35:dbl, element #2=w34:dbl)  [unwired: 2 in]
  n163 = Index Array(array=w37) -> (element #1=w33:dbl, element #2=w32:dbl)  [unwired: 2 in]
  n164 = Build Array(w35, w34, w33, w32) -> (w29:dbl[])
  n165 = Array Size(array=w25) -> (size(s)=w31:i32[])
  n166 = Index Array(array=w31) -> (element=w30:i32)  [unwired: 1 in]
  n167 = Insert Into Array(array=w25, index (row)=w30, new element=w29) -> (→"Start End Points RRT":dbl[][])  [unwired: 1 in]
